vi "GPIB Send.vi"(8 "error in (no error)":errorcluster, 9 "text":string, 10 "address":i16, 11 "id":i32) -> (0 "error out":errorcluster, 1 "text out":string, 3 "function return":u32)   [LabVIEW 2014, in "atmcd32d.lvlib"]
doc: "unsigned int WINAPI GPIBSend(int id, short address, char * text);"
uses:
  atmcd32d.lvlib
  atmcd32d.dll
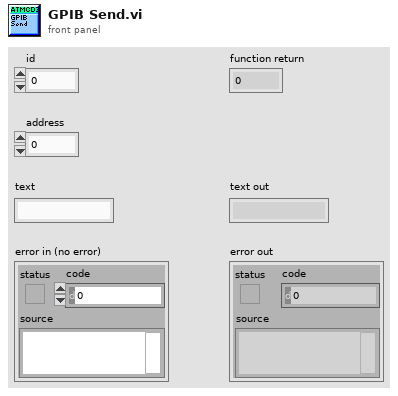
[diagram p1: front panel]
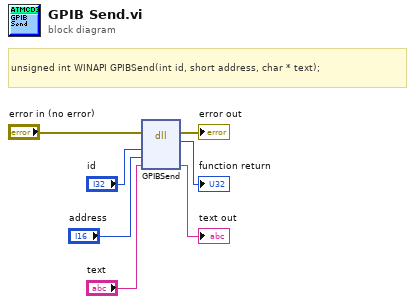
[diagram p0: block diagram]
diagram:
  # "unsigned int WINAPI GPIBSend(int id, short address, char * text);"
  n1 = dll-call lib="C:/Users/Bakir/Documents/Lambda2-Testing/lib/Andorlib/atmcd32d.*" fn="GPIBSend"(error in="error in (no error)", "id"="id", "address"="address", "text"="text") -> (error out=→"error out":errorcluster, →"function return":u32, "text"=→"text out":string)  [unwired: 4 in, 1 out]
